vi "Read X-Axis Data Measurement Points.vi"(7 "Channel (1)":i32=1, 8 "error in (no error)":errorcluster, 11 "VISA resource name":refnum<visa-resource-name>) -> (0 "error out":errorcluster, 2 "X-Axis Data Measurement Points":dbl[](array[numeric]), 3 "VISA resource name out":refnum<visa-resource-name>)   [LabVIEW 2018, in "Agilent ENA Series.lvlib"]
doc: "Reads out the data of measurement points of X axis, for selected channel."
uses:
  Agilent ENA Series.lvlib
panel:
  out "size(s)":i32
  in  "Trace":i32
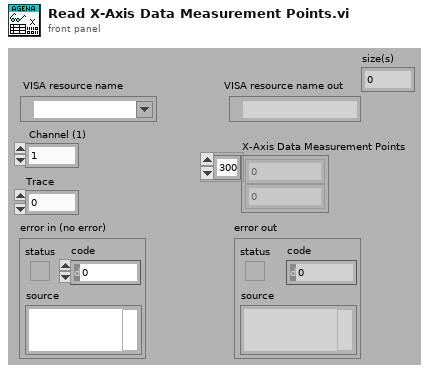
[diagram p1: front panel]
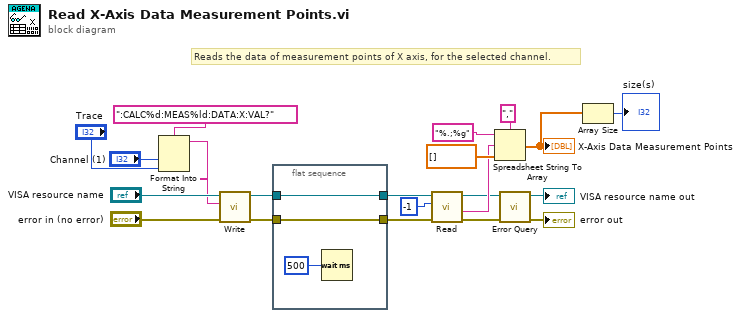
[diagram p0: block diagram]
diagram:
  # "Reads the data of measurement points of X axis, for the selected channel."
  n1 = Format Into String(format string=":CALC%d:MEAS%ld:DATA:X:VAL?", "Channel (1)", "Trace") -> (resulting string=w3:string)  [unwired: 2 in, 1 out]
  n2 = call "Write.vi"("error in (no error)"="error in (no error)", "String ()"=w3, "VISA resource name"="VISA resource name") -> ("error out"=w13:errorcluster, "VISA resource name out"=w14:refnum<visa-resource-name>)  [unwired: 6 in, 1 out]
  n3 = flat-sequence {
    tunnel: w14 -> [w22]
    tunnel: w13 -> [w24]
    tunnel: [w24] -> w11
    tunnel: [w22] -> w12
    frame #0 {
      n4 = Wait (ms)(milliseconds to wait=u32 500) -> ()  [unwired: 1 out]
    }
  }
  n5 = call "Read.vi"("error in (no error)"=w11, "Number Of Bytes"=-1, "VISA resource name"=w12) -> ("error out"=w8:errorcluster, "String"=w16:string, "VISA resource name out"=w10:refnum<visa-resource-name>)  [unwired: 5 in, 1 out]
  n6 = Spreadsheet String To Array(delimiter (Tab)=",", format string="%.;%g", spreadsheet string=w16, array type (2D Dbl)=dbl[] []) -> (array=w2:dbl[])
  "X-Axis Data Measurement Points" <- w2
  n7 = call "Error Query.vi"("error in (no error)"=w8, "VISA resource name"=w10) -> ("error out"=→"error out":errorcluster, "VISA resource name out"=→"VISA resource name out":refnum<visa-resource-name>)  [unwired: 6 in, 2 out]
  n8 = Array Size(array=w2) -> (size(s)=→"size(s)":i32)
